vi "Update UI.vi"(8 "error in (no error)":errorcluster, 11 "Main Display in":refnum<class "Main Display.lvclass">) -> (0 "error out":errorcluster, 3 "Main Display out":refnum<class "Main Display.lvclass">)   [LabVIEW 2016, in "Assert API Components.lvlib" / "Assert Display.lvlib" / "Main Display.lvlib" / "Main Display.lvclass"]
doc: "Builds the packet of information (assert data and colours) to send to the UI"
uses:
  Main Display.lvclass
  Main Display.lvclass/Main Display.ctl
  Display Configurations/Base Display Configuration.lvclass
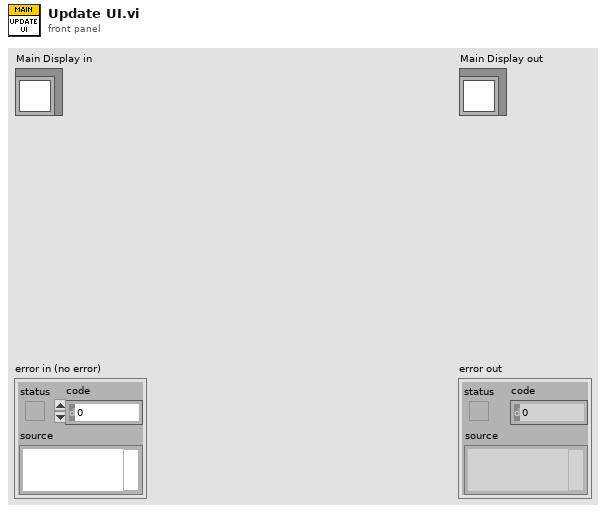
[diagram p1: front panel]
types:
  T1 = typedef "Assert API Components.lvlib/Assert Display.lvlib/Main Display.lvlib/Display Data.ctl" = cluster{"ItemNames":string[][], "Pass Fail Status":bool[], "Display Colours":T2, "Assert VI UID Array":i32[]}
  T2 = typedef "Assert API Components.lvlib/Assert Display.lvlib/Main Display.lvlib/Display Colours.ctl" = cluster{"Enable Colours":bool, "Passed Colour":u32, "Failed Colour":u32}
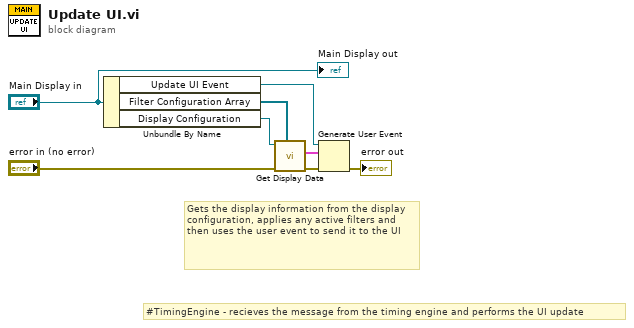
[diagram p0: block diagram]
diagram:
  # "#TimingEngine - recieves the message from the timing engine and performs the UI update"
  # "Gets the display information from the display configuration, applies any active filters and then uses the user event to send it to the UI"
  n1 = Unbundle By Name("Main Display in") -> ("Update UI Event"=w5:refnum<user-event>, "Filter Configuration Array"=w1:refnum<class "Base Filter.lvclass">[], "Display Configuration"=w2:refnum<class "Base Display Configuration.lvclass">)
  n2 = call-dynamic "Get Display Data.vi"("Filter Configuration Array"=w1, "error in (no error)"="error in (no error)", "Base Display Configuration in"=w2) -> ("error out"=w4:errorcluster, "Display Data"=w3:T1)  [unwired: 7 in]
  n3 = Generate User Event(user event=w5, event data cluster=w3, error in=w4) -> (error out=→"error out":errorcluster)  [unwired: 1 in, 1 out]
  "Main Display out" <- "Main Display in"
